vi "Detekce_pruchodu_nulami.vi"(2 "Citlivost vypoctu frekvence":i32, 3 "dt 2":dbl format="%#_13g", 4 "array":dbl[](array[numeric])) -> (0 "Pole indexu pruchodu nulou":i32[](array[numeric]), 1 "Numeric":dbl)   [LabVIEW 2019]
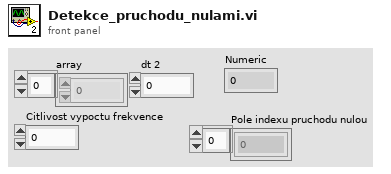
[diagram p1: front panel]
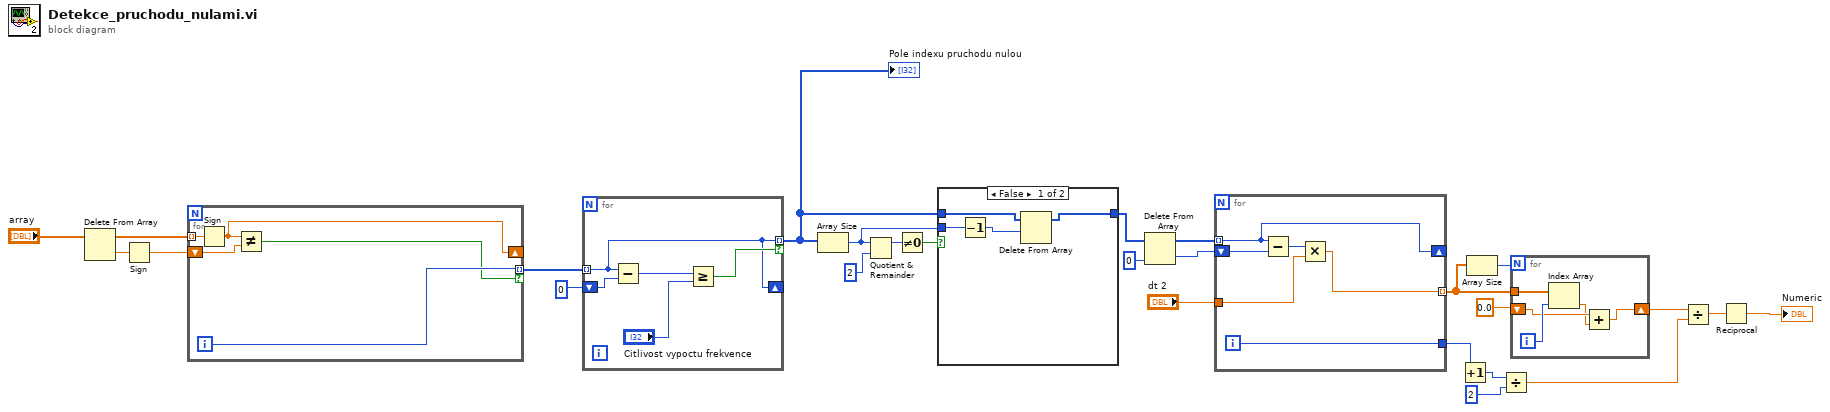
[diagram p0: block diagram]
diagram:
  n1 = Delete From Array(array="array") -> (deleted portion=w24:dbl, array with subset deleted=w26:dbl[])  [unwired: 2 in]
  n2 = Sign(1:w24) -> (0:w23:dbl)
  n3 = for {
    tunnel: w26 -> [w31] mode=indexing
    shift-right: [w27] -> _
    shift-left: w23 -> [w30]
    tunnel: [w29] -> w22 mode=indexing if=w28
    i -> [w29]
    n4 = Sign(1:w31) -> (0:w27:dbl)
    n5 = Not Equal?(x=w27, y=w30) -> (x != y?=w28:bool)
  }
  n6 = for {
    tunnel: w22 -> [w32] mode=indexing
    shift-right: [w32] -> _
    shift-left: 0 -> [w36]
    tunnel: [w32] -> w13 mode=indexing if=w33
    n7 = Subtract(x=w32, y=w36) -> (x-y=w35:i32)
    n8 = Greater Or Equal?(x=w35, y="Citlivost vypoctu frekvence") -> (x >= y?=w33:bool)
  }
  "Pole indexu pruchodu nulou" <- w13
  n9 = Array Size(array=w13) -> (size(s)=w11:i32)
  n10 = Quotient & Remainder(x=w11, y=2) -> (x-y*floor(x/y)=w15:i32)  [unwired: 1 out]
  n11 = Not Equal To 0?(x=w15) -> (x != 0?=w14:bool)
  n12 = case shown="False" w14 {
    tunnel: w13 -> [w40 w41]
    tunnel: [w37 w41] -> w12
    tunnel: w11 -> [w39 _]
    frame False {
      n13 = Decrement(x=w39) -> (x-1=w38:i32)
      n14 = Delete From Array(array=w40, length=w38) -> (array with subset deleted=w37:i32[])  [unwired: 1 in, 1 out]
    }
    frame True {
    }
  }
  n15 = Delete From Array(array=w12, index=0) -> (deleted portion=w19:i32, array with subset deleted=w20:i32[])  [unwired: 1 in]
  n16 = for {
    tunnel: w20 -> [w44] mode=indexing
    shift-right: [w44] -> _
    shift-left: w19 -> [w47]
    tunnel: "dt 2" -> [w46]
    tunnel: [w43] -> w17
    tunnel: [w42] -> w9 mode=indexing
    i -> [w43]
    n17 = Subtract(x=w44, y=w47) -> (x-y=w45:i32)
    n18 = Multiply(x=w45, y=w46) -> (x*y=w42:dbl)
  }
  n19 = Increment(x=w17) -> (x+1=w6:i32)
  n20 = Array Size(array=w9) -> (size(s)=w8:i32)
  n21 = Divide(x=w6, y=2) -> (x/y=w4:dbl)
  n22 = for {
    N: w8 -> [_]
    tunnel: w9 -> [w52]
    shift-right: [w48] -> w3
    shift-left: 0.0 -> [w50]
    i -> [w51]
    n23 = Index Array(array=w52, index=w51) -> (element=w49:dbl)
    n24 = Add(x=w50, y=w49) -> (x+y=w48:dbl)
  }
  n25 = Divide(x=w3, y=w4) -> (x/y=w2:dbl)
  n26 = Reciprocal(x=w2) -> (1/x=→"Numeric":dbl)
